vi "Exo1.vi"() -> ()   [LabVIEW 2018]
panel:
  in  "Y":u8 max=9 step=1
  out "X/Y":dbl
  out "X*Y":dbl
  out "X-Y":dbl
  out "X+Y":dbl
  in  "X":u8 max=9
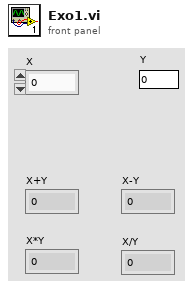
[diagram p1: front panel]
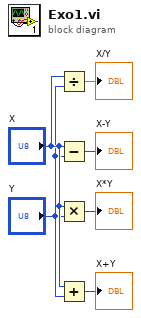
[diagram p0: block diagram]
diagram:
  n1 = Divide(x="X", y="Y") -> (x/y=→"X/Y":dbl)
  n2 = Subtract(x="X", y="Y") -> (x-y=→"X-Y":u8)
  n3 = Multiply(x="X", y="Y") -> (x*y=→"X*Y":u8)
  n4 = Add(x="X", y="Y") -> (x+y=→"X+Y":u8)
